vi "Add Child Node w Attr.vi"(4 "Values":string[](array[string]), 6 "Names":string[](array[string]), 8 "Error In":errorcluster, 9 "Tag Name":string, 10 "Parent Node":refnum<k20>, 11 "DOM In":refnum<k20>) -> (0 "Error Out":errorcluster, 1 "Child Node":refnum<k20>, 2 "Parent Node":refnum<k20>, 3 "DOM Out":refnum<k20>)   [LabVIEW 2020, in "UIM.lvlib" / "UIM.lvclass"]
uses:
  UIM.lvclass
  <resource>/objmgr/DOMUserDefRef.rc
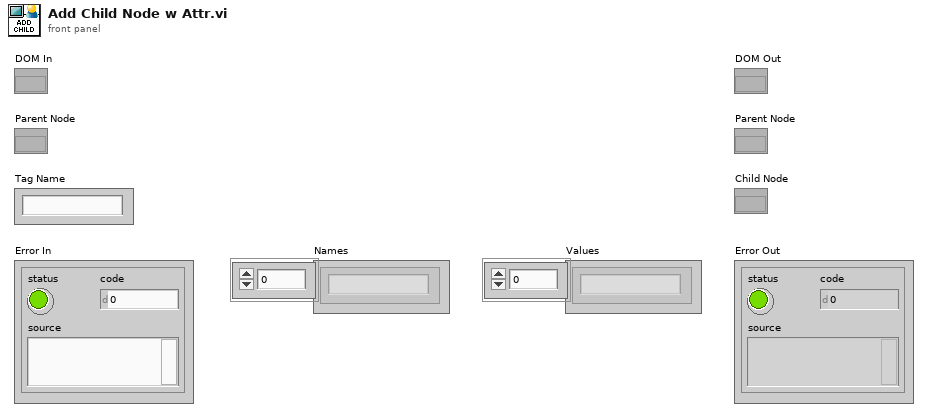
[diagram p1: front panel]
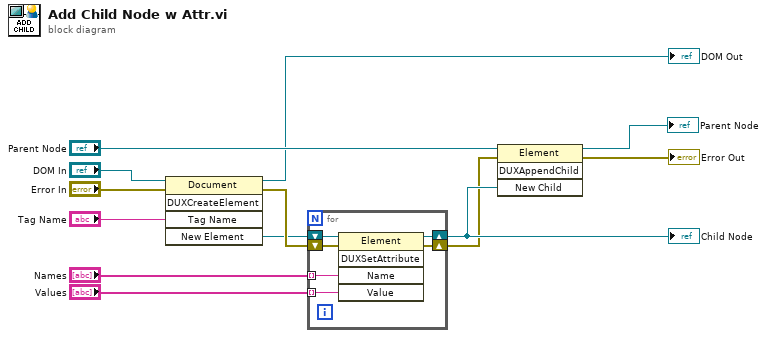
[diagram p0: block diagram]
diagram:
  n1 = invoke class="Document" method="DUXCreateElement"(reference="DOM In", error in="Error In", "Tag Name"="Tag Name") -> (reference out=→"DOM Out":refnum<k20>, error out=w9:errorcluster, "New Element"=w6:refnum<k20>)  [unwired: 2 in, 2 out]
  n2 = for {
    tunnel: "Names" -> [w18] mode=indexing
    tunnel: "Values" -> [w17] mode=indexing
    shift-right: [w16] -> w13
    shift-left: w6 -> [w19]
    shift-right: [w14] -> w11
    shift-left: w9 -> [w15]
    n3 = invoke class="Element" method="DUXSetAttribute"(reference=w19, error in=w15, "Name"=w18, "Value"=w17) -> (reference out=w16:refnum<k20>, error out=w14:errorcluster)  [unwired: 1 in, 3 out]
  }
  "Child Node" <- w13
  n4 = invoke class="Element" method="DUXAppendChild"(reference="Parent Node", error in=w11, "New Child"=w13) -> (reference out=→"Parent Node":refnum<k20>, error out=→"Error Out":errorcluster)  [unwired: 1 in, 2 out]
